vi "Choose MM Setpoint.vi"(8 "Right Encoder Pos":i32, 9 "\"Done with step\" enough":bool, 10 "Steps":T1, 11 "Left Encoder Pos":i32) -> (0 "Right Motor Setpoint":dbl, 1 "MM on last step":bool, 2 "Index of Current Step":dbl, 3 "Left Motor Setpoint":dbl)   [LabVIEW 2018]
uses:
  Drive Motion Magic Setpoints.ctl
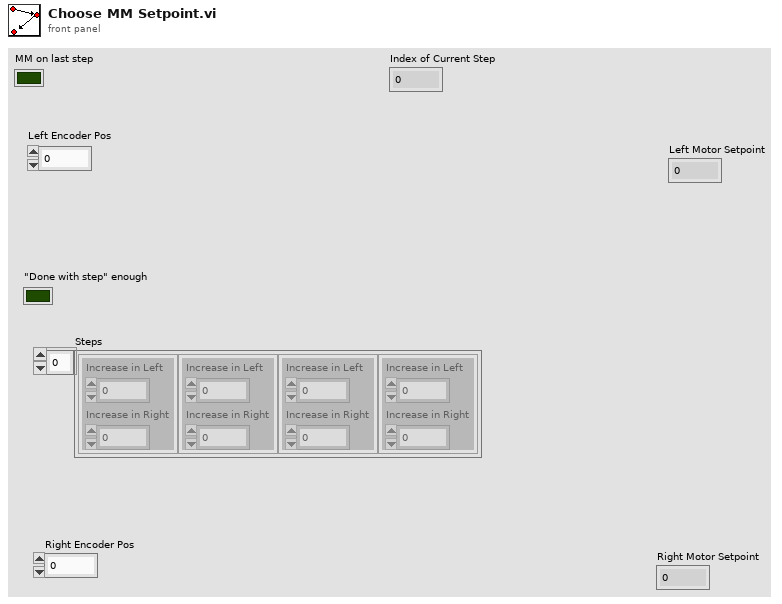
[diagram p1: front panel]
types:
  T1 = typedef "Drive Motion Magic Setpoints.ctl" = cluster{"Increase in Left":dbl, "Increase in Right":dbl}[]
  T2 = cluster{"Increase in Left":dbl, "Increase in Right":dbl}
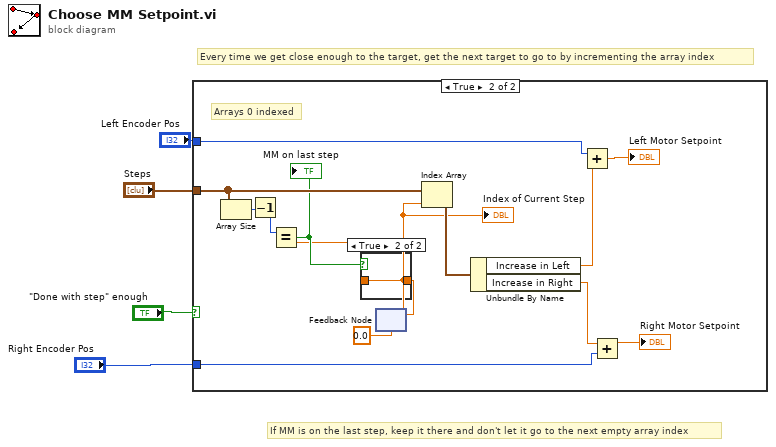
[diagram p0: block diagram]
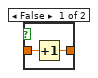
[diagram p3: hidden frame]
diagram:
  # "Every time we get close enough to the target, get the next target to go to by incrementing the array index"
  # "If MM is on the last step, keep it there and don't let it go to the next empty array index"
  n1 = case shown="True" "\"Done with step\" enough" {
    tunnel: "Steps" -> [_ w13]
    tunnel: "Left Encoder Pos" -> [_ w16]
    tunnel: "Right Encoder Pos" -> [_ w14]
    frame False {
    }
    frame True {
      # "Arrays 0 indexed"
      n2 = Array Size(array=w13) -> (size(s)=w7:i32)
      n3 = Decrement(x=w7) -> (x-1=w6:i32)
      n4 = feedback #1(0.0) -> (w5:dbl)
      "Index of Current Step" <- w5
      n5 = Equal?(x=w6, y=w5) -> (x = y?=w9:bool)
      "MM on last step" <- w9
      n6 = case shown="True" w9 {
        tunnel: [w20 w21] -> w8
        tunnel: w5 -> [w19 w21]
        frame False {
          n7 = Increment(x=w19) -> (x+1=w20:dbl)
        }
        frame True {
        }
      }
      n8 = feedback-in #1(w8) -> ()
      n9 = Index Array(array=w13, index=w5) -> (element=w18:T2)
      n10 = Unbundle By Name(w18) -> ("Increase in Left"=w17:dbl, "Increase in Right"=w15:dbl)
      n11 = Add(x=w16, y=w17) -> (x+y=→"Left Motor Setpoint":dbl)
      n12 = Add(x=w15, y=w14) -> (x+y=→"Right Motor Setpoint":dbl)
    }
  }
